vi "C-to-F.vi"() -> ()   [LabVIEW 2017]
panel:
  out "Waveform Chart":dbl(graph)
  in  "stop":bool
  out "Celsius":dbl(slide) scale=-50.0..100.0
  in  "Fahrenheit":dbl(slide) scale=-20.0..200.0
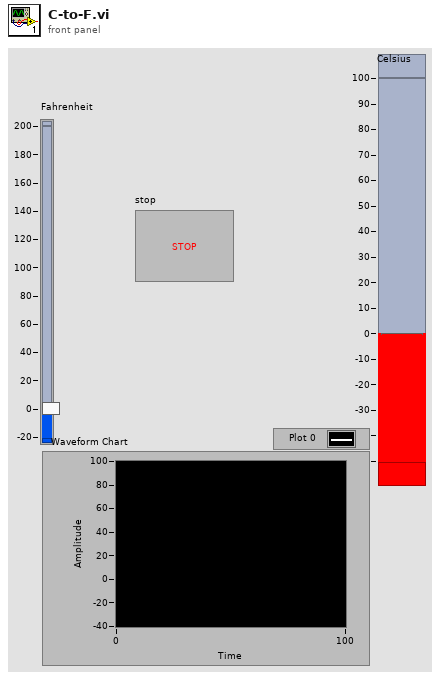
[diagram p1: front panel]
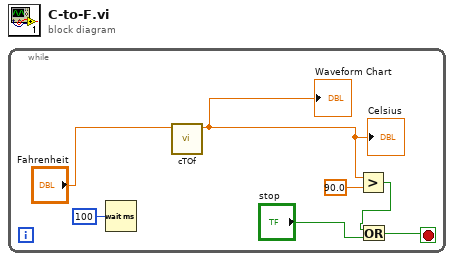
[diagram p0: block diagram]
diagram:
  n1 = while {
    stop <- w3 stop-if-true
    n2 = Wait (ms)(milliseconds to wait=u32 100) -> ()  [unwired: 1 out]
    n3 = call "cTOf.vi"("Fahrenheit"="Fahrenheit") -> ("Numeric"=w2:dbl)  [unwired: 10 in]
    "Celsius" <- w2
    "Waveform Chart" <- w2
    n4 = Greater?(x=w2, y=90.0) -> (0:w4:bool)
    n5 = Or(x=w4, y="stop") -> (x .or. y?=w3:bool)
  }
